vi "Load and Build.vi"(0 "Project Path":path, 1 "Data String (\"\")":string, 5 "Report Folder":path, 7 "Build Config Override":path, 9 "Project Build Class Name (Empty = \"Project Builder\")":string, 11 "error in (no error)":errorcluster) -> (4 "Project Builder out":refnum<class "Project Builder.lvclass">, 10 "Success?":bool, 15 "error out":errorcluster)   [LabVIEW 2020, in "ProjectBuilder.lvlib"]
doc: "Load and populate a 'Project Builder'-class and call the Build Project.vi method on the loaded class."
uses:
  ProjectBuilder.lvlib
  Class/Project Builder/Project Builder.lvclass
  Class/Project Builder/Project Builder.lvclass/Project Builder.ctl
  <vilib>/Utility/error.llb/Error Cluster From Error Code.vi
  <vilib>/ErrorRing/Error Ring.xnode
  PPL/HDH.ClassLoader.lvlibp
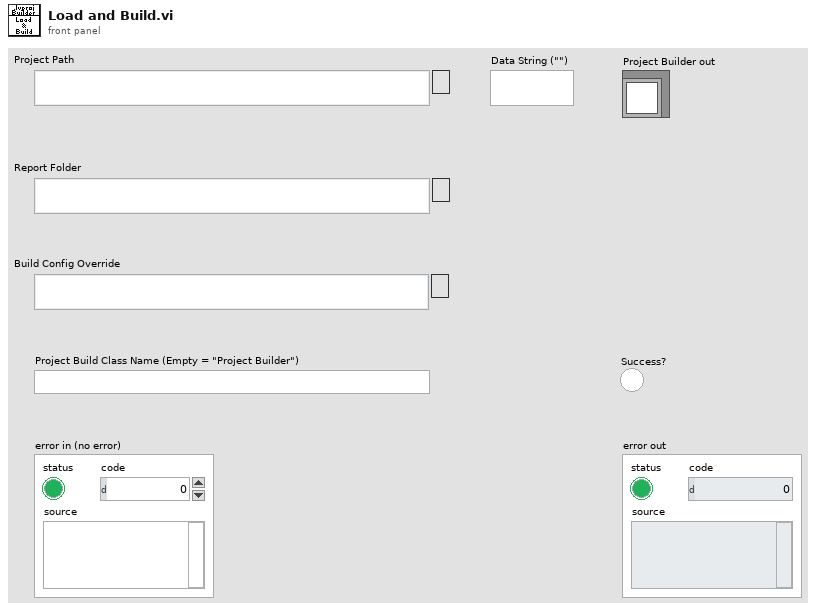
[diagram p1: front panel]
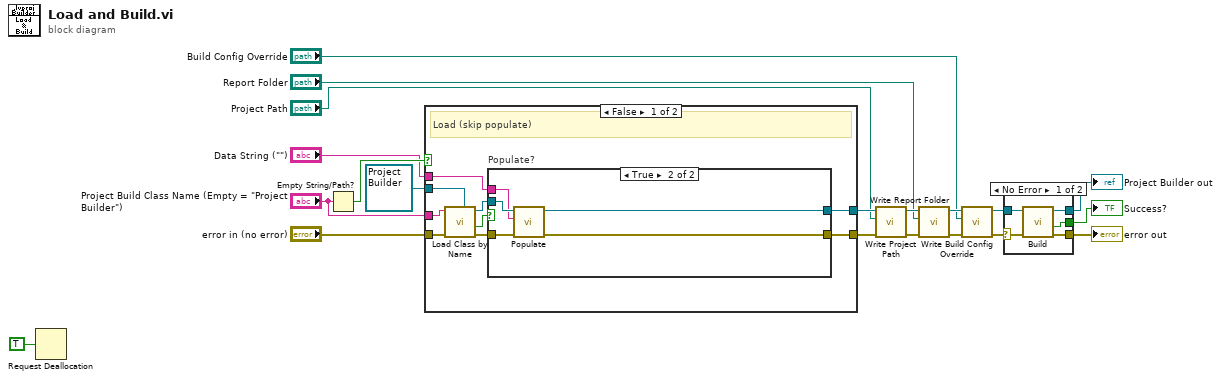
[diagram p0: block diagram]
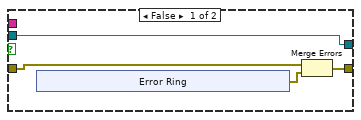
[diagram p3: hidden frame]
diagram:
  n1 = Request Deallocation(TRUE ("flag")) -> ()
  n2 = Empty String/Path?(string/path="Project Build Class Name (Empty = \"Project Builder\")") -> (empty?=w20:bool)
  n3 = case shown="False" w20 {
    tunnel: "Project Build Class Name (Empty = \"Project Builder\")" -> [w29 _]
    tunnel: "error in (no error)" -> [w28 w43]
    tunnel: refnum<class "Project Builder.lvclass"> refnum ("ProjectBuilder.lvlib:Project Builder.lvclass") -> [w27 w44]
    tunnel: [w25 w44] -> w15
    tunnel: [w23 w43] -> w11
    tunnel: "Data String (\"\")" -> [w22 _]
    frame False {
      # "Load (skip populate)"
      n4 = call "Load Class by Name.vi"("Class Type"=w27, "error in (no error)"=w28, "Base Class Name"=w29) -> ("error out"=w24:errorcluster, "Load and Type Success?"=w21:bool, "Loaded Class"=w26:refnum<class "Project Builder.lvclass">)  [unwired: 5 in, 1 out]
      n5 = case "Populate?" shown="True" w21 {
        tunnel: w26 -> [w33 w42]
        tunnel: [w33 w41] -> w25
        tunnel: w24 -> [w31 w40]
        tunnel: [w30 w39] -> w23
        tunnel: w22 -> [_ w38]
        frame False {
          n6 = xnode "Error Ring"() -> ("error out"=w32:errorcluster)
          n7 = Merge Errors(w31, w32) -> (w30:errorcluster)
        }
        frame True {
          n8 = call-dynamic "Populate.vi"("error in (no error)"=w40, "Data String"=w38, "Project Builder in"=w42) -> ("error out"=w39:errorcluster, "Project Builder out"=w41:refnum<class "Project Builder.lvclass">)  [unwired: 7 in]
        }
      }
    }
    frame True {
      # "Use parent (don't populate)"
    }
  }
  n9 = call "Write Project Path.vi"("error in (no error)"=w11, "Project Path"="Project Path", "Project Builder in"=w15) -> ("error out"=w10:errorcluster, "Project Builder out"=w14:refnum<class "Project Builder.lvclass">)  [unwired: 7 in]
  n10 = call "Write Report Folder.vi"("error in (no error)"=w10, "Report Folder"="Report Folder", "Project Builder in"=w14) -> ("error out"=w9:errorcluster, "Project Builder out"=w3:refnum<class "Project Builder.lvclass">)  [unwired: 7 in]
  n11 = call "Write Build Config Override.vi"("error in (no error)"=w9, "Build Config Override"="Build Config Override", "Project Builder in"=w3) -> ("error out"=w4:errorcluster, "Project Builder out"=w2:refnum<class "Project Builder.lvclass">)  [unwired: 7 in]
  n12 = case shown="No Error" w4 {
    selector: w4 -> [w48 w51]
    tunnel: w2 -> [w49 w50]
    tunnel: [w47 w51] -> w8
    tunnel: [w46 _] -> w7
    tunnel: [w45 w50] -> w6
    frame No Error {
      n13 = call "Build.vi"("error in (no error)"=w48, "Project Builder in"=w49) -> ("error out"=w47:errorcluster, "Success?"=w46:bool, "Project Builder out"=w45:refnum<class "Project Builder.lvclass">)  [unwired: 7 in]
    }
    frame Error {
    }
  }
  "error out" <- w8
  "Success?" <- w7
  "Project Builder out" <- w6
